vi "Test for AUTO.vi"(8 "error in":errorcluster, 11 "VISA resource name":refnum<visa-resource-name>) -> (0 "error out":errorcluster, 3 "VISA resource name out":refnum<visa-resource-name>)   [LabVIEW 2011, in "GPT-9000.lvlib"]
uses:
  <instrlib>/GPT-9000/GPT-9000.lvlib
panel:
  in  "New Test name":string
  in  "RENAME":bool
  in  "Query Error":bool
  out "Error Message":string
  in  "SWAP":bool
  in  "Destination Step":u8=1 min=1 max=16
  in  "Source Step":u8=1 min=1 max=16
  in  "SKIP":bool
  in  "Setup the Skip Step Status":u8(ring) items=["OFF", "ON"]
  in  "Select Step for Skip":u8=1 min=1 max=16
  in  "DEL":bool
  in  "Selected the Step to Deletes":u8=1 min=1 max=16
  in  "ADD":bool
  in  "Selected the MANU test Step to ADD":u8=1 min=1 max=100
  in  "Move":bool
  in  "Desired Destination Step":u8=1 min=1 max=16
  in  "Source Step":u8=1 min=1 max=16
  out "End Step":u8
  out "Str16":string
  out "Str15":string
  out "Str14":string
  out "Str13":string
  out "Str12":string
  out "Str11":string
  out "Str10":string
  out "Str9":string
  out "Str8":string
  out "Str7":string
  out "Str6":string
  out "Str5":string
  out "Str4":string
  out "Str3":string
  out "Str2":string
  out "Str1":string
  out "Step":u8
  out "S16":bool
  out "S15":bool
  out "S14":bool
  out "S13":bool
  out "S12":bool
  out "S11":bool
  out "S10":bool
  out "S9":bool
  out "S8":bool
  out "S7":bool
  out "S6":bool
  out "S5":bool
  out "S4":bool
  out "S3":bool
  out "S2":bool
  out "S1":bool
  out "(Num:Step)":string[](array[string])
  out "Return the test name":string
  in  "Start":bool
  in  "Stop":bool
  in  "Test number":u8 min=1 max=100
  in  "Configure RS232 Baud Rate":u32(ring)=9600 items=["9600"=9600, "19200"=19200, "38400"=38400, "57600"=57600, "115200"=115200]
  out "ID Return String":string
  in  "Clear Error(True)":bool=TRUE
  in  "ID Query (True)":bool=TRUE
  # "Test for Auto Mode"
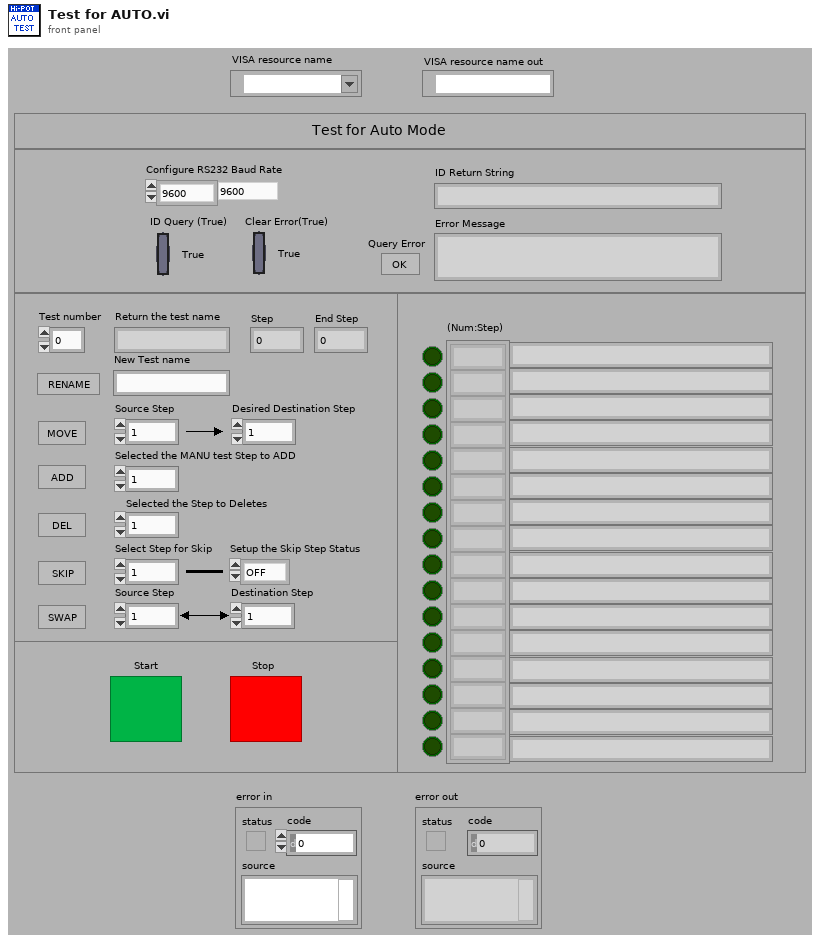
[diagram p1: front panel]
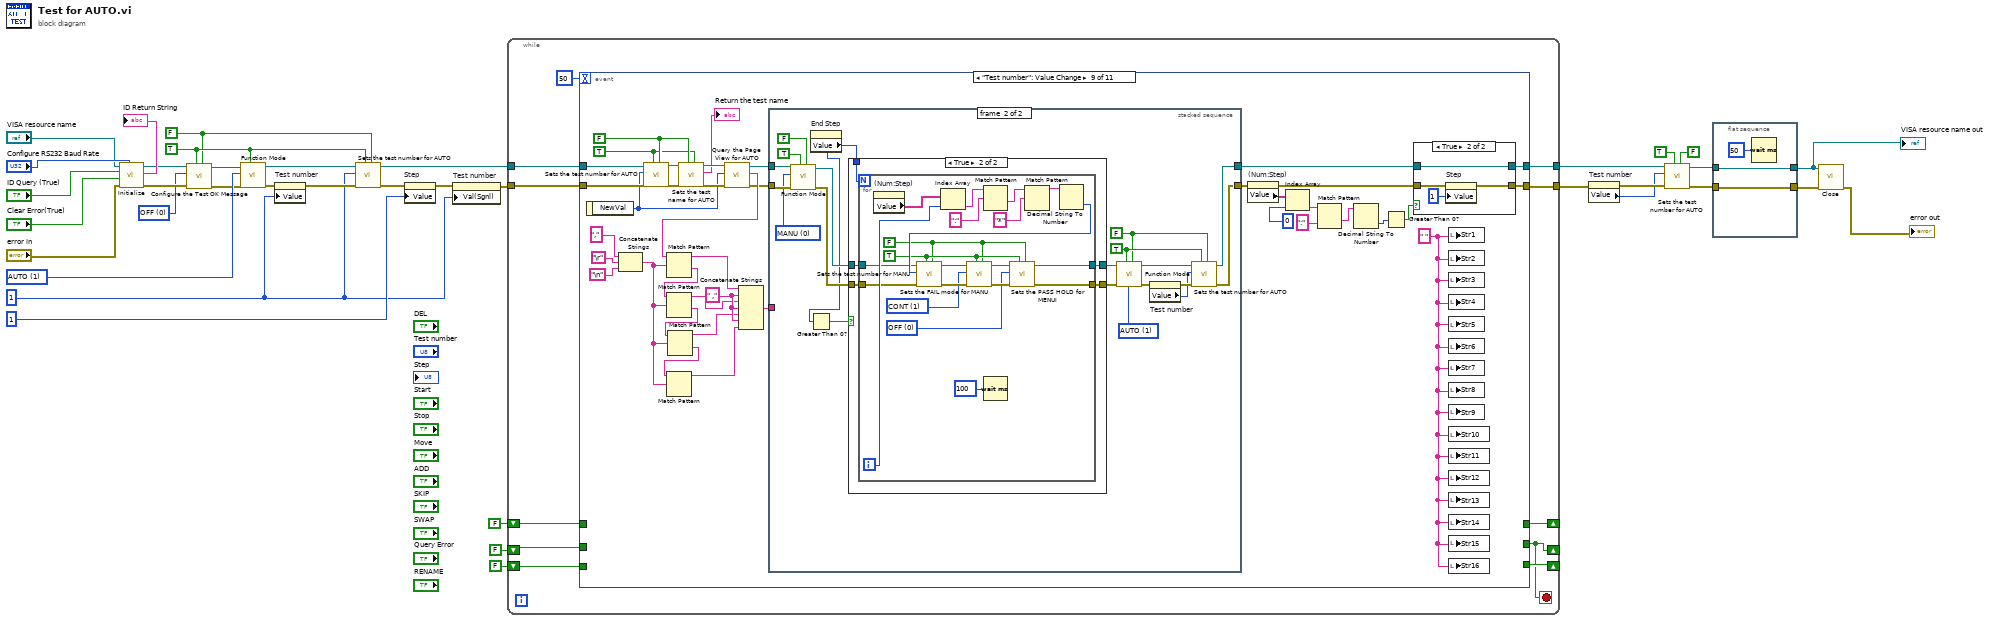
[diagram p0: block diagram]
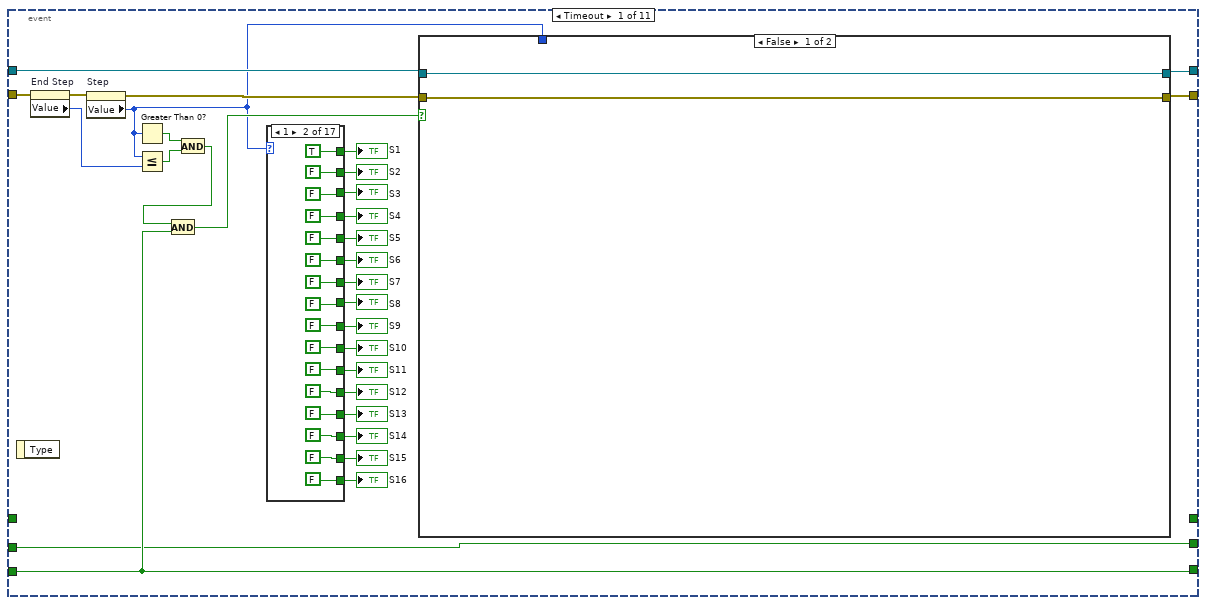
[diagram p2: hidden frame]
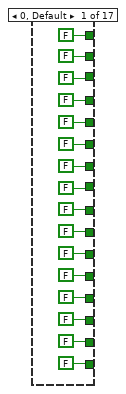
[diagram p3: hidden frame]
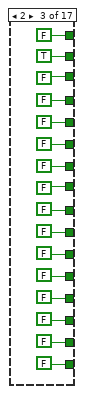
[diagram p4: hidden frame]
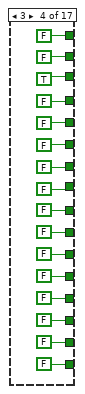
[diagram p5: hidden frame]
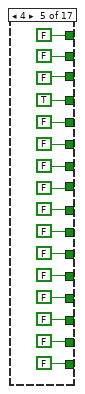
[diagram p6: hidden frame]
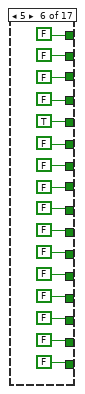
[diagram p7: hidden frame]
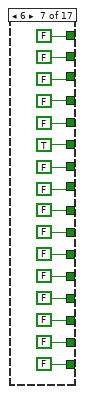
[diagram p8: hidden frame]
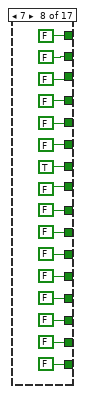
[diagram p9: hidden frame]
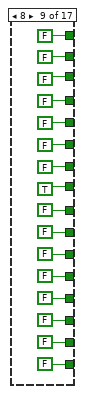
[diagram p10: hidden frame]
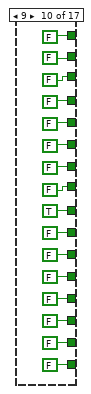
[diagram p11: hidden frame]
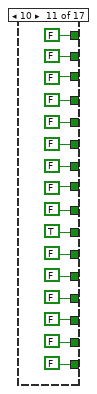
[diagram p12: hidden frame]
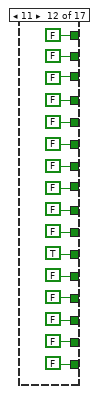
[diagram p13: hidden frame]
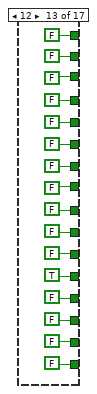
[diagram p14: hidden frame]
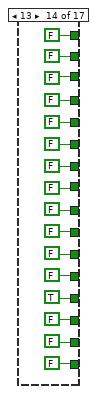
[diagram p15: hidden frame]
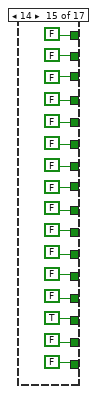
[diagram p16: hidden frame]
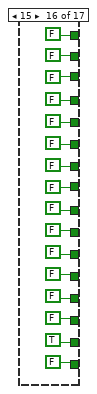
[diagram p17: hidden frame]
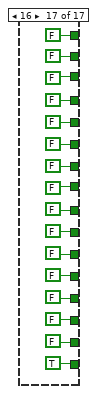
[diagram p18: hidden frame]
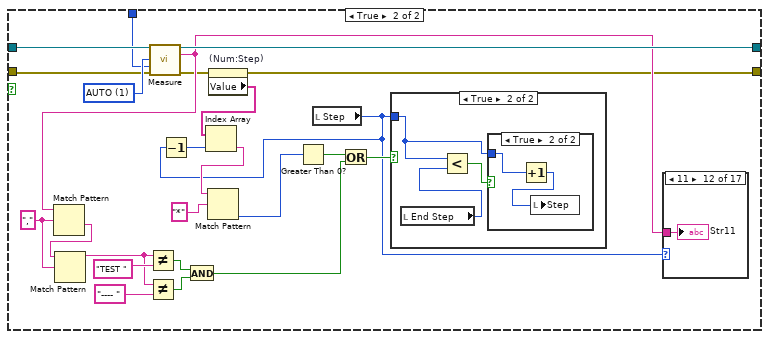
[diagram p19: hidden frame]
diagram:
  w3 = u8 0 items=["OFF", "ON"] ("Send Message when test stop")
  w22 = u8 1 ("Test number")
  w31 = u8 1 items=["AUTO"=1, "MANU"=0] ("Function Mode")
  w1 = FALSE ("Enable to Query")
  w2 = TRUE
  n1 = call <instrlib>:"Initialize.vi"("Configure RS232 Baud Rate"="Configure RS232 Baud Rate", "error in (no error)"="error in", "Clear Error(True)"="Clear Error(True)", "ID Query (True)"="ID Query (True)", "VISA resource name"="VISA resource name") -> ("error out"=w5:errorcluster, "ID Return String"=→"ID Return String":string, "VISA resource name out"=w7:refnum<visa-resource-name>)  [unwired: 3 in, 1 out]
  n2 = call <instrlib>:"Configure the Test OK Message.vi"("Query the Message"=w1, "Setup the Message"=w2, "error in"=w5, "Send Message when test stop"=w3, "VISA resource name"=w7) -> ("error out"=w4:errorcluster, "VISA resource name out"=w6:refnum<visa-resource-name>)  [unwired: 4 in, 1 out]
  n3 = call <instrlib>:"Function Mode.vi"("Enable to Setup"=w2, "error in"=w4, "Function Mode"=w31, "VISA resource name"=w6) -> ("error out"=w27:errorcluster, "VISA resource name out"=w24:refnum<visa-resource-name>)  [unwired: 5 in, 1 out]
  n4 = property on="Test number" class="DigNum (strict)"(error in=w27, "Value"=w22) -> (error out=w23:errorcluster)  [unwired: 1 in, 1 out]
  n5 = call <instrlib>:"Sets the test number for AUTO.vi"("Enable to Query"=w1, "Enable to Setup"=w2, "error in"=w23, "Test number"=w22, "VISA resource name"=w24) -> ("error out"=w12:errorcluster, "VISA resource name out"=w13:refnum<visa-resource-name>)  [unwired: 4 in, 1 out]
  n6 = property on="Step" class="DigNum (strict)"(error in=w12, "Value"=u8 1 ("Step")) -> (error out=w26:errorcluster)  [unwired: 1 in, 1 out]
  n7 = property on="Test number" class="DigNum (strict)"(error in=w26, "Val(Sgnl)"=w22) -> (error out=w25:errorcluster)  [unwired: 1 in, 1 out]
  n8 = while {
    tunnel: w13 -> [w45]
    tunnel: w25 -> [w44]
    tunnel: [w48] -> w19
    tunnel: [w47] -> w16
    shift-right: [w46] -> _
    shift-left: FALSE -> [w43]
    shift-right: [w39] -> _
    shift-left: FALSE -> [w42]
    shift-right: [w41] -> _
    shift-left: FALSE -> [w40]
    stop <- w39 stop-if-true
    n9 = event shown="[8] \"Test number\": Value Change" {
      selector: _ -> [_ _ _ _ _ _ _ _ _ _ _]
      dyn-events: _ -> [_ _ _ _ _ _ _ _ _ _ _]
      timeout: 50 -> [_ _ _ _ _ _ _ _ _ _ _]
      tunnel: [w74 w403 w421 w441 w460 w479 w494 w511 w538 w651 w675] -> w48
      tunnel: [w71 w402 w420 w440 w459 w478 w493 w510 w536 w650 w674] -> w47
      tunnel: w45 -> [w78 w405 w423 w443 w462 w481 w496 w514 w557 w653 w676]
      tunnel: w44 -> [w51 w404 w422 w442 w461 w480 w495 w513 w556 w652 w668]
      tunnel: w43 -> [w75 w398 w417 w436 w455 w474 w489 w512 _ w648 w671]
      tunnel: [w75 w398 w417 w436 w455 w474 w489 w512 _ _ w672] -> w46
      tunnel: w42 -> [w49 _ _ _ _ _ _ _ _ w649 w673]
      tunnel: [w49 _ _ _ _ _ _ _ _ w646 _] -> w39
      tunnel: [_ _ _ _ _ _ _ _ _ w645 _] -> w41
      tunnel: w40 -> [_ _ _ _ _ _ _ _ _ w644 _]
      event Timeout {
        n10 = event-data() -> ()  [unwired: 1 in, 1 out]
        n11 = property on="End Step" class="DigNum (strict)"(error in=w51) -> (error out=w53:errorcluster, "Value"=w52:u8)  [unwired: 1 in, 1 out]
        n12 = property on="Step" class="DigNum (strict)"(error in=w53) -> (error out=w77:errorcluster, "Value"=w50:u8)  [unwired: 1 in, 1 out]
        n13 = Greater Than 0?(x=w50) -> (x > 0?=w72:bool)
        n14 = Less Or Equal?(x=w50, y=w52) -> (x <= y?=w73:bool)
        n15 = And(x=w72, y=w73) -> (x .and. y?=w54:bool)
        n16 = And(x=w54, y=w75) -> (x .and. y?=w76:bool)
        n17 = case shown="1" w50 {
          tunnel: [FALSE TRUE FALSE FALSE FALSE FALSE FALSE FALSE FALSE FALSE FALSE FALSE FALSE FALSE FALSE FALSE FALSE] -> w70
          tunnel: [FALSE FALSE TRUE FALSE FALSE FALSE FALSE FALSE FALSE FALSE FALSE FALSE FALSE FALSE FALSE FALSE FALSE] -> w69
          tunnel: [FALSE FALSE FALSE TRUE FALSE FALSE FALSE FALSE FALSE FALSE FALSE FALSE FALSE FALSE FALSE FALSE FALSE] -> w68
          tunnel: [FALSE FALSE FALSE FALSE FALSE TRUE FALSE FALSE FALSE FALSE FALSE FALSE FALSE FALSE FALSE FALSE FALSE] -> w67
          tunnel: [FALSE FALSE FALSE FALSE FALSE FALSE FALSE TRUE FALSE FALSE FALSE FALSE FALSE FALSE FALSE FALSE FALSE] -> w66
          tunnel: [FALSE FALSE FALSE FALSE FALSE FALSE FALSE FALSE TRUE FALSE FALSE FALSE FALSE FALSE FALSE FALSE FALSE] -> w65
          tunnel: [FALSE FALSE FALSE FALSE FALSE FALSE FALSE FALSE FALSE TRUE FALSE FALSE FALSE FALSE FALSE FALSE FALSE] -> w64
          tunnel: [FALSE FALSE FALSE FALSE FALSE FALSE FALSE FALSE FALSE FALSE TRUE FALSE FALSE FALSE FALSE FALSE FALSE] -> w63
          tunnel: [FALSE FALSE FALSE FALSE FALSE FALSE FALSE FALSE FALSE FALSE FALSE TRUE FALSE FALSE FALSE FALSE FALSE] -> w62
          tunnel: [FALSE FALSE FALSE FALSE FALSE FALSE FALSE FALSE FALSE FALSE FALSE FALSE TRUE FALSE FALSE FALSE FALSE] -> w61
          tunnel: [FALSE FALSE FALSE FALSE FALSE FALSE FALSE FALSE FALSE FALSE FALSE FALSE FALSE TRUE FALSE FALSE FALSE] -> w60
          tunnel: [FALSE FALSE FALSE FALSE FALSE FALSE FALSE FALSE FALSE FALSE FALSE FALSE FALSE FALSE TRUE FALSE FALSE] -> w59
          tunnel: [FALSE FALSE FALSE FALSE FALSE FALSE FALSE FALSE FALSE FALSE FALSE FALSE FALSE FALSE FALSE TRUE FALSE] -> w58
          tunnel: [FALSE FALSE FALSE FALSE FALSE FALSE FALSE FALSE FALSE FALSE FALSE FALSE FALSE FALSE FALSE FALSE TRUE] -> w57
          tunnel: [FALSE FALSE FALSE FALSE TRUE FALSE FALSE FALSE FALSE FALSE FALSE FALSE FALSE FALSE FALSE FALSE FALSE] -> w56
          tunnel: [FALSE FALSE FALSE FALSE FALSE FALSE TRUE FALSE FALSE FALSE FALSE FALSE FALSE FALSE FALSE FALSE FALSE] -> w55
          frame 0, Default {
          }
          frame 1 {
          }
          frame 2 {
          }
          frame 3 {
          }
          frame 4 {
          }
          frame 5 {
          }
          frame 6 {
          }
          frame 7 {
          }
          frame 8 {
          }
          frame 9 {
          }
          frame 10 {
          }
          frame 11 {
          }
          frame 12 {
          }
          frame 13 {
          }
          frame 14 {
          }
          frame 15 {
          }
          frame 16 {
          }
        }
        "S1" <- w70
        "S2" <- w69
        "S3" <- w68
        "S4" <- w56
        "S5" <- w67
        "S6" <- w55
        "S7" <- w66
        "S8" <- w65
        "S9" <- w64
        "S10" <- w63
        "S11" <- w62
        "S12" <- w61
        "S13" <- w60
        "S14" <- w59
        "S15" <- w58
        "S16" <- w57
        n18 = case shown="False" w76 {
          tunnel: w78 -> [w352 w375]
          tunnel: w77 -> [w351 w361]
          tunnel: [w352 w374] -> w74
          tunnel: [w351 w359] -> w71
          tunnel: w50 -> [_ w366]
          frame False {
          }
          frame True {
            w372 = "," ("regular expression")
            w376 = u8 1 items=["MANU", "AUTO"] ("Function Mode Numeric")
            n19 = call <instrlib>:"Measure.vi"("VISA resource name"=w375, "Function Mode Numeric"=w376, "Step number for Auto Mode"=w366, "error in"=w361) -> ("VISA resource name out"=w374:refnum<visa-resource-name>, "Return  the test status"=w367:string, "error out"=w360:errorcluster)  [unwired: 8 in, 1 out]
            n20 = Match Pattern(string=w367, regular expression=w372) -> (after substring=w373:string)  [unwired: 1 in, 3 out]
            n21 = Match Pattern(string=w373, regular expression=w372) -> (before substring=w353:string)  [unwired: 1 in, 3 out]
            n22 = Not Equal?(x=w353, y="TEST ") -> (x != y?=w369:bool)
            n23 = Not Equal?(x=w353, y="---- ") -> (x != y?=w368:bool)
            n24 = And(x=w369, y=w368) -> (x .and. y?=w358:bool)
            n25 = property on="(Num:Step)" class="Arr (strict)"(error in=w360) -> (error out=w359:errorcluster, "Value"=w356:string[])  [unwired: 1 in, 1 out]
            n26 = local read "Step"() -> (w354:u8)
            n27 = Decrement(x=w354) -> (x-1=w355:u8)
            n28 = Index Array(array=w356, index=w355) -> (element=w364:string)
            n29 = Match Pattern(string=w364, regular expression="*") -> (offset past match=w363:i32)  [unwired: 1 in, 3 out]
            n30 = Greater Than 0?(x=w363) -> (x > 0?=w357:bool)
            n31 = Or(x=w357, y=w358) -> (x .or. y?=w362:bool)
            n32 = case shown="True" w362 {
              tunnel: w354 -> [_ w394]
              frame False {
              }
              frame True {
                n33 = local read "End Step"() -> (w393:u8)
                n34 = Less?(x=w394, y=w393) -> (x < y?=w395:bool)
                n35 = case shown="True" w395 {
                  tunnel: w394 -> [_ w396]
                  frame False {
                  }
                  frame True {
                    n36 = Increment(x=w396) -> (x+1=w397:u8)
                    n37 = local write "Step"(w397) -> ()
                  }
                }
              }
            }
            n38 = case shown="11" w354 {
              tunnel: w367 -> [_ w377 w378 w379 w380 w381 w382 w383 w384 w385 w386 w387 w388 w389 w390 w391 w392]
              frame 0, Default {
              }
              frame 1 {
                "Str1" <- w377
              }
              frame 2 {
                "Str2" <- w378
              }
              frame 3 {
                "Str3" <- w379
              }
              frame 4 {
                "Str4" <- w380
              }
              frame 5 {
                "Str5" <- w381
              }
              frame 6 {
                "Str6" <- w382
              }
              frame 7 {
                "Str7" <- w383
              }
              frame 8 {
                "Str8" <- w384
              }
              frame 9 {
                "Str9" <- w385
              }
              frame 10 {
                "Str10" <- w386
              }
              frame 11 {
                "Str11" <- w387
              }
              frame 12 {
                "Str12" <- w388
              }
              frame 13 {
                "Str13" <- w389
              }
              frame 14 {
                "Str14" <- w390
              }
              frame 15 {
                "Str15" <- w391
              }
              frame 16 {
                "Str16" <- w392
              }
            }
          }
        }
      }
      event "DEL": Value Change {
        n39 = event-data() -> ("NewVal"=w399:bool)  [unwired: 1 in]
        n40 = Not(x=w398) -> (.not. x?=w400:bool)
        n41 = And(x=w399, y=w400) -> (x .and. y?=w401:bool)
        n42 = case shown="True" w401 {
          tunnel: w405 -> [w407 w414]
          tunnel: w404 -> [w406 w413]
          tunnel: [w406 w410] -> w402
          tunnel: [w407 w409] -> w403
          frame False {
          }
          frame True {
            n43 = call <instrlib>:"Deletes the selected step for AUTO.vi"("error in"=w413, "Selected the Step to Deletes"="Selected the Step to Deletes", "VISA resource name"=w414) -> ("error out"=w412:errorcluster, "VISA resource name out"=w409:refnum<visa-resource-name>)  [unwired: 7 in]
            n44 = property on="Test number" class="DigNum (strict)"(error in=w412) -> (error out=w411:errorcluster, "Value"=w408:u8)  [unwired: 1 in, 1 out]
            n45 = property on="Test number" class="DigNum (strict)"(error in=w411, "Val(Sgnl)"=w408) -> (error out=w410:errorcluster)  [unwired: 1 in, 1 out]
          }
        }
      }
      event "RENAME": Value Change {
        n46 = event-data() -> ("NewVal"=w418:bool)  [unwired: 1 in]
        n47 = Not(x=w417) -> (.not. x?=w416:bool)
        n48 = And(x=w418, y=w416) -> (x .and. y?=w419:bool)
        n49 = case shown="True" w419 {
          tunnel: w423 -> [w425 w434]
          tunnel: w422 -> [w424 w433]
          tunnel: [w425 w432] -> w421
          tunnel: [w424 w427] -> w420
          frame False {
          }
          frame True {
            n50 = call <instrlib>:"Sets the test name for AUTO.vi"("Enable to Query"=FALSE, "Enable to Setup"=TRUE, "error in"=w433, "Test name"="New Test name", "VISA resource name"=w434) -> ("error out"=w429:errorcluster, "VISA resource name out"=w432:refnum<visa-resource-name>)  [unwired: 4 in, 1 out]
            n51 = property on="Test number" class="DigNum (strict)"(error in=w429) -> (error out=w428:errorcluster, "Value"=w426:u8)  [unwired: 1 in, 1 out]
            n52 = property on="Test number" class="DigNum (strict)"(error in=w428, "Val(Sgnl)"=w426) -> (error out=w427:errorcluster)  [unwired: 1 in, 1 out]
          }
        }
      }
      event "SWAP": Value Change {
        n53 = event-data() -> ("NewVal"=w438:bool)  [unwired: 1 in]
        n54 = Not(x=w436) -> (.not. x?=w437:bool)
        n55 = And(x=w438, y=w437) -> (x .and. y?=w439:bool)
        n56 = case shown="True" w439 {
          tunnel: w443 -> [w445 w452]
          tunnel: w442 -> [w444 w451]
          tunnel: [w445 w450] -> w441
          tunnel: [w444 w447] -> w440
          frame False {
          }
          frame True {
            n57 = call <instrlib>:"Swaps the source step with destination step for AUTO.vi"("error in"=w451, "Destination Step"="Destination Step", "Source Step"="Source Step", "VISA resource name"=w452) -> ("error out"=w449:errorcluster, "VISA resource name out"=w450:refnum<visa-resource-name>)  [unwired: 6 in]
            n58 = property on="Test number" class="DigNum (strict)"(error in=w449) -> (error out=w448:errorcluster, "Value"=w446:u8)  [unwired: 1 in, 1 out]
            n59 = property on="Test number" class="DigNum (strict)"(error in=w448, "Val(Sgnl)"=w446) -> (error out=w447:errorcluster)  [unwired: 1 in, 1 out]
          }
        }
      }
      event "SKIP": Value Change {
        n60 = event-data() -> ("NewVal"=w457:bool)  [unwired: 1 in]
        n61 = Not(x=w455) -> (.not. x?=w456:bool)
        n62 = And(x=w457, y=w456) -> (x .and. y?=w458:bool)
        n63 = case shown="True" w458 {
          tunnel: w462 -> [w464 w471]
          tunnel: w461 -> [w463 w470]
          tunnel: [w463 w467] -> w459
          tunnel: [w464 w466] -> w460
          frame False {
          }
          frame True {
            n64 = call <instrlib>:"Skips the selected step for AUTO.vi"("error in"=w470, "Setup the Skip Step Status"="Setup the Skip Step Status", "Select Step for Skip"="Select Step for Skip", "VISA resource name"=w471) -> ("error out"=w469:errorcluster, "VISA resource name out"=w466:refnum<visa-resource-name>)  [unwired: 6 in]
            n65 = property on="Test number" class="DigNum (strict)"(error in=w469) -> (error out=w468:errorcluster, "Value"=w465:u8)  [unwired: 1 in, 1 out]
            n66 = property on="Test number" class="DigNum (strict)"(error in=w468, "Val(Sgnl)"=w465) -> (error out=w467:errorcluster)  [unwired: 1 in, 1 out]
          }
        }
      }
      event "Query Error": Value Change {
        n67 = event-data() -> ("NewVal"=w477:bool)  [unwired: 1 in]
        n68 = Not(x=w474) -> (.not. x?=w475:bool)
        n69 = And(x=w477, y=w475) -> (x .and. y?=w476:bool)
        n70 = case shown="True" w476 {
          tunnel: w481 -> [w483 w487]
          tunnel: w480 -> [w482 w486]
          tunnel: [w483 w485] -> w479
          tunnel: [w482 w484] -> w478
          frame False {
          }
          frame True {
            n71 = call <instrlib>:"Error Query.vi"("error in (no error)"=w486, "VISA resource name"=w487) -> ("error out"=w484:errorcluster, "Error Message"=→"Error Message":string, "VISA resource name out"=w485:refnum<visa-resource-name>)  [unwired: 6 in, 1 out]
          }
        }
      }
      event "ADD": Value Change {
        n72 = event-data() -> ("NewVal"=w491:bool)  [unwired: 1 in]
        n73 = Not(x=w489) -> (.not. x?=w490:bool)
        n74 = And(x=w491, y=w490) -> (x .and. y?=w492:bool)
        n75 = case shown="True" w492 {
          tunnel: w496 -> [w498 w505]
          tunnel: [w498 w504] -> w494
          tunnel: w495 -> [w497 w503]
          tunnel: [w497 w499] -> w493
          frame False {
          }
          frame True {
            n76 = call <instrlib>:"Add the selected MANU test step for AUTO.vi"("error in"=w503, "Selected the MANU test Step to ADD"="Selected the MANU test Step to ADD", "VISA resource name"=w505) -> ("error out"=w502:errorcluster, "VISA resource name out"=w504:refnum<visa-resource-name>)  [unwired: 7 in]
            n77 = property on="Test number" class="DigNum (strict)"(error in=w502) -> (error out=w501:errorcluster, "Value"=w500:u8)  [unwired: 1 in, 1 out]
            n78 = property on="Test number" class="DigNum (strict)"(error in=w501, "Val(Sgnl)"=w500) -> (error out=w499:errorcluster)  [unwired: 1 in, 1 out]
          }
        }
      }
      event "Move": Value Change {
        n79 = event-data() -> ("NewVal"=w508:bool)  [unwired: 1 in]
        n80 = Not(x=w512) -> (.not. x?=w507:bool)
        n81 = And(x=w508, y=w507) -> (x .and. y?=w509:bool)
        n82 = case shown="True" w509 {
          tunnel: w514 -> [w516 w523]
          tunnel: w513 -> [w515 w522]
          tunnel: [w516 w521] -> w511
          tunnel: [w515 w518] -> w510
          frame False {
          }
          frame True {
            n83 = call <instrlib>:"Moves the Source step to the desired destination for AUTO.vi"("error in"=w522, "Desired Destination Step"="Desired Destination Step", "Source Step"="Source Step", "VISA resource name"=w523) -> ("error out"=w520:errorcluster, "VISA resource name out"=w521:refnum<visa-resource-name>)  [unwired: 6 in]
            n84 = property on="Test number" class="DigNum (strict)"(error in=w520) -> (error out=w519:errorcluster, "Value"=w517:u8)  [unwired: 1 in, 1 out]
            n85 = property on="Test number" class="DigNum (strict)"(error in=w519, "Val(Sgnl)"=w517) -> (error out=w518:errorcluster)  [unwired: 1 in, 1 out]
          }
        }
      }
      event "Test number": Value Change {
        w533 = " " ("Str1")
        w547 = " ," ("string")
        w562 = FALSE ("Enable to Query")
        w561 = TRUE
        n86 = event-data() -> ("NewVal"=w555:u8)  [unwired: 1 in]
        n87 = Concatenate Strings("," ("string"), "\r" ("string"), "\n" ("string")) -> (w551:string)
        n88 = call <instrlib>:"Sets the test number for AUTO.vi"("Enable to Query"=w562, "Enable to Setup"=w561, "error in"=w556, "Test number"=w555, "VISA resource name"=w557) -> ("error out"=w563:errorcluster, "VISA resource name out"=w564:refnum<visa-resource-name>)  [unwired: 4 in, 1 out]
        n89 = call <instrlib>:"Sets the test name for AUTO.vi"("Enable to Query"=w561, "Enable to Setup"=w562, "error in"=w563, "VISA resource name"=w564) -> ("error out"=w559:errorcluster, "Return the test name"=→"Return the test name":string, "VISA resource name out"=w560:refnum<visa-resource-name>)  [unwired: 5 in]
        n90 = call <instrlib>:"Query the Page View for AUTO.vi"("error in"=w559, "Manual test number of Page View"=w555, "VISA resource name"=w560) -> ("error out"=w531:errorcluster, "Return the Page View String"=w554:string, "VISA resource name out"=w530:refnum<visa-resource-name>)  [unwired: 5 in, 1 out]
        n91 = Match Pattern(string=w554, regular expression=w551) -> (before substring=w546:string, after substring=w550:string)  [unwired: 1 in, 2 out]
        n92 = Match Pattern(string=w550, regular expression=w551) -> (before substring=w545:string, after substring=w549:string)  [unwired: 1 in, 2 out]
        n93 = Match Pattern(string=w549, regular expression=w551) -> (before substring=w544:string, after substring=w548:string)  [unwired: 1 in, 2 out]
        n94 = Match Pattern(string=w548, regular expression=w551) -> (before substring=w543:string)  [unwired: 1 in, 3 out]
        n95 = Concatenate Strings(w546, w547, w545, w547, w544, w547, w543) -> (w542:string)
        n96 = stacked-sequence {
          tunnel: w542 -> [w566 _]
          tunnel: w531 -> [_ w594]
          tunnel: w530 -> [_ w597]
          tunnel: [_ w605] -> w529
          tunnel: [_ w604] -> w528
          frame #0 {
            n97 = for {
              N: 16 -> [_]
              tunnel: w566 -> [w583]
              tunnel: [w580] -> w565 mode=indexing
              i -> [w578]
              n98 = Equal To 0?(x=w578) -> (x = 0?=w574:bool)
              n99 = Increment(x=w578) -> (x+1=w570:i32)
              n100 = feedback #1() -> (w581:string)  [unwired: 1 in]
              n101 = Select(t=w583, s=w574, f=w581) -> (s? t:f=w584:string)
              n102 = Match Pattern(string=w584, regular expression=",") -> (before substring=w580:string, after substring=w582:string)  [unwired: 1 in, 2 out]
              n103 = feedback-in #1(w582) -> ()
              n104 = Match Pattern(string=w580, regular expression=":") -> (after substring=w577:string)  [unwired: 1 in, 3 out]
              n105 = Decimal String To Number(string=w577) -> (number=w576:i32)  [unwired: 2 in, 1 out]
              n106 = Greater Than 0?(x=w576) -> (x > 0?=w572:bool)
              n107 = Equal To 0?(x=w576) -> (x = 0?=w573:bool)
              n108 = And(x=w573, y=w574) -> (x .and. y?=w568:bool)
              n109 = Select(t=0, s=w568, f=w570) -> (s? t:f=w571:i32)
              n110 = Or(x=w572, y=w568) -> (x .or. y?=w575:bool)
              n111 = case shown="True" w575 {
                tunnel: w571 -> [_ w586]
                frame False {
                }
                frame True {
                  "End Step" <- w586
                }
              }
            }
            "(Num:Step)" <- w565
          }
          frame #1 {
            w593 = u8 0 items=["AUTO"=1, "MANU"=0] ("Function Mode")
            w598 = u8 1 items=["AUTO"=1, "MANU"=0] ("Function Mode")
            w591 = FALSE ("Enable to Query")
            w592 = TRUE ("Enable to Setup")
            n112 = call <instrlib>:"Function Mode.vi"("Enable to Query"=FALSE, "Enable to Setup"=TRUE, "error in"=w594, "Function Mode"=w593, "VISA resource name"=w597) -> ("error out"=w595:errorcluster, "VISA resource name out"=w596:refnum<visa-resource-name>)  [unwired: 4 in, 1 out]
            n113 = property on="End Step" class="DigNum (strict)"() -> ("Value"=w587:u8)  [unwired: 2 in, 2 out]
            n114 = Greater Than 0?(x=w587) -> (x > 0?=w588:bool)
            n115 = case shown="True" w588 {
              tunnel: [w608 w613] -> w602
              tunnel: [w607 w612] -> w599
              tunnel: w596 -> [w608 w611]
              tunnel: w595 -> [w607 w610]
              tunnel: w587 -> [_ w609]
              frame False {
              }
              frame True {
                n116 = for {
                  N: w609 -> [_]
                  tunnel: w611 -> [w622]
                  tunnel: w610 -> [w621]
                  tunnel: [w616] -> w613
                  tunnel: [w615] -> w612
                  i -> [w634]
                  w619 = u8 1 items=["STOP", "CONT", "HOLD"] ("FAIL mode Setting")
                  w620 = u8 0 items=["OFF", "ON"] ("PASS HOLD Setting")
                  w617 = FALSE ("Enable to Query")
                  w618 = TRUE ("Enable to Setup")
                  n117 = property on="(Num:Step)" class="Arr (strict)"() -> ("Value"=w633:string[])  [unwired: 2 in, 2 out]
                  n118 = Index Array(array=w633, index=w634) -> (element=w629:string)
                  n119 = Match Pattern(string=w629, regular expression=":") -> (after substring=w628:string)  [unwired: 1 in, 3 out]
                  n120 = Wait (ms)(milliseconds to wait=u32 100) -> ()  [unwired: 1 out]
                  n121 = Match Pattern(string=w628, regular expression="*") -> (before substring=w630:string)  [unwired: 1 in, 3 out]
                  n122 = Decimal String To Number(string=w630) -> (number=w623:i32)  [unwired: 2 in, 1 out]
                  n123 = call <instrlib>:"Sets the test number for MANU.vi"("Enable to Query"=w617, "Enable to Setup"=w618, "error in"=w621, "Test number"=w623, "VISA resource name"=w622) -> ("error out"=w624:errorcluster, "VISA resource name out"=w625:refnum<visa-resource-name>)  [unwired: 4 in, 1 out]
                  n124 = call <instrlib>:"Sets the FAIL mode for MANU.vi"("Enable to Query the FAIL mode"=w617, "Enable to Setup the FAIL mode"=w618, "error in"=w624, "FAIL mode Setting"=w619, "VISA resource name"=w625) -> ("error out"=w627:errorcluster, "VISA resource name out"=w626:refnum<visa-resource-name>)  [unwired: 4 in, 1 out]
                  n125 = call <instrlib>:"Sets the PASS HOLD for MENUI.vi"("Enable to Query the PASS HOLD"=w617, "Enable to Setup the PASS HOLD"=w618, "error in"=w627, "PASS HOLD Setting"=w620, "VISA resource name"=w626) -> ("error out"=w615:errorcluster, "VISA resource name out"=w616:refnum<visa-resource-name>)  [unwired: 4 in, 1 out]
                }
              }
            }
            n126 = call <instrlib>:"Function Mode.vi"("Enable to Query"=w591, "Enable to Setup"=w592, "error in"=w599, "Function Mode"=w598, "VISA resource name"=w602) -> ("error out"=w600:errorcluster, "VISA resource name out"=w601:refnum<visa-resource-name>)  [unwired: 4 in, 1 out]
            n127 = property on="Test number" class="DigNum (strict)"(error in=w600) -> (error out=w606:errorcluster, "Value"=w603:u8)  [unwired: 1 in, 1 out]
            n128 = call <instrlib>:"Sets the test number for AUTO.vi"("Enable to Query"=w591, "Enable to Setup"=w592, "error in"=w606, "Test number"=w603, "VISA resource name"=w601) -> ("error out"=w604:errorcluster, "VISA resource name out"=w605:refnum<visa-resource-name>)  [unwired: 4 in, 1 out]
          }
        }
        n129 = property on="(Num:Step)" class="Arr (strict)"(error in=w528) -> (error out=w527:errorcluster, "Value"=w526:string[])  [unwired: 1 in, 1 out]
        n130 = Index Array(array=w526, index=0) -> (element=w540:string)
        n131 = Match Pattern(string=w540, regular expression=":") -> (after substring=w535:string)  [unwired: 1 in, 3 out]
        n132 = Decimal String To Number(string=w535) -> (number=w534:i32)  [unwired: 2 in, 1 out]
        n133 = Greater Than 0?(x=w534) -> (x > 0?=w537:bool)
        n134 = case shown="True" w537 {
          tunnel: [w638 w642] -> w538
          tunnel: w529 -> [w638 w642]
          tunnel: w527 -> [w637 w641]
          tunnel: [w636 w640] -> w536
          frame False {
            n135 = property on="Step" class="DigNum (strict)"(error in=w637, "Value"=u8 0 ("Numeric")) -> (error out=w636:errorcluster)  [unwired: 1 in, 1 out]
          }
          frame True {
            n136 = property on="Step" class="DigNum (strict)"(error in=w641, "Value"=u8 1 ("Numeric")) -> (error out=w640:errorcluster)  [unwired: 1 in, 1 out]
          }
        }
        n137 = local write "Str1"(w533) -> ()
        n138 = local write "Str2"(w533) -> ()
        n139 = local write "Str3"(w533) -> ()
        n140 = local write "Str4"(w533) -> ()
        n141 = local write "Str5"(w533) -> ()
        n142 = local write "Str6"(w533) -> ()
        n143 = local write "Str7"(w533) -> ()
        n144 = local write "Str8"(w533) -> ()
        n145 = local write "Str9"(w533) -> ()
        n146 = local write "Str10"(w533) -> ()
        n147 = local write "Str11"(w533) -> ()
        n148 = local write "Str12"(w533) -> ()
        n149 = local write "Str13"(w533) -> ()
        n150 = local write "Str14"(w533) -> ()
        n151 = local write "Str15"(w533) -> ()
        n152 = local write "Str16"(w533) -> ()
      }
      event "Stop": Mouse Down {
        w643 = TRUE ("x")
        n153 = event-data() -> ()  [unwired: 1 in, 1 out]
        n154 = And(x=w643, y=w648) -> (x .and. y?=w647:bool)
        n155 = case shown="True" w647 {
          tunnel: w653 -> [w655 w659]
          tunnel: w652 -> [w654 w658]
          tunnel: [w655 w657] -> w651
          tunnel: [w654 w656] -> w650
          frame False {
          }
          frame True {
            w662 = u8 0 items=["OFF", "ON"] ("Function Test")
            n156 = call <instrlib>:"Function Test.vi"("VISA resource name"=w659, "Function Test"=w662, "error in"=w658, "Enable to Setup"=TRUE, "Enable to Query"=FALSE) -> ("VISA resource name out"=w657:refnum<visa-resource-name>, "error out"=w656:errorcluster)  [unwired: 3 in, 1 out]
          }
        }
        n157 = Or(x=w643, y=w644) -> (x .or. y?=w645:bool)
        n158 = Or(x=w647, y=w649) -> (x .or. y?=w646:bool)
      }
      event "Start": Mouse Down {
        n159 = event-data() -> ()  [unwired: 1 in, 1 out]
        n160 = Not(x=w671) -> (.not. x?=w670:bool)
        n161 = property on="End Step" class="DigNum (strict)"(error in=w668) -> (error out=w667:errorcluster, "Value"=w666:u8)  [unwired: 1 in, 1 out]
        n162 = Not(x=w673) -> (.not. x?=w669:bool)
        n163 = And(x=w670, y=w669) -> (x .and. y?=w664:bool)
        n164 = Greater Than 0?(x=w666) -> (x > 0?=w665:bool)
        n165 = And(x=w665, y=w664) -> (x .and. y?=w663:bool)
        n166 = Or(x=w663, y=w671) -> (x .or. y?=w672:bool)
        n167 = case shown="False" w663 {
          tunnel: w676 -> [w677 w685]
          tunnel: w667 -> [w678 w684]
          tunnel: [w677 w680] -> w675
          tunnel: [w678 w679] -> w674
          frame False {
          }
          frame True {
            w683 = u8 1 items=["OFF", "ON"] ("Function Test")
            n168 = call <instrlib>:"Function Test.vi"("VISA resource name"=w685, "Function Test"=w683, "error in"=w684, "Enable to Setup"=TRUE, "Enable to Query"=FALSE) -> ("VISA resource name out"=w680:refnum<visa-resource-name>, "error out"=w679:errorcluster)  [unwired: 3 in, 1 out]
          }
        }
      }
    }
  }
  n169 = property on="Test number" class="DigNum (strict)"(error in=w16) -> (error out=w15:errorcluster, "Value"=w14:u8)  [unwired: 1 in, 1 out]
  n170 = call <instrlib>:"Sets the test number for AUTO.vi"("Enable to Query"=FALSE, "Enable to Setup"=TRUE, "error in"=w15, "Test number"=w14, "VISA resource name"=w19) -> ("error out"=w17:errorcluster, "VISA resource name out"=w18:refnum<visa-resource-name>)  [unwired: 4 in, 1 out]
  n171 = flat-sequence {
    tunnel: w18 -> [w687]
    tunnel: [w687] -> w9
    tunnel: w17 -> [w686]
    tunnel: [w686] -> w11
    frame #0 {
      n172 = Wait (ms)(milliseconds to wait=u32 50) -> ()  [unwired: 1 out]
    }
  }
  n173 = call <instrlib>:"Close.vi"("error in (no error)"=w11, "VISA resource name"=w9) -> ("error out"=→"error out":errorcluster)  [unwired: 9 in]
  "VISA resource name out" <- w9
